vi "EOL All-Station AI Debug Buffer.vi"(5 "number of stations":i32=4, 7 "station idx":i32=4, 8 "Data to Write (Ch-Ro, Samp-Col)":sgl[][](array[numeric]) format="%.2f", 9 "Buffer Size (seconds/2500)":i32=5000, 11 "Mode":enum16{"Initialize", "Read", "Write"}(ring)=enum."Read") -> (2 "Data Read (Samp-Ro, Ch-Col)":sgl[][](array[numeric]) format="%.2f")   [LabVIEW 2018]
doc: "This VI is used in many locations throughout the program as a data buffer. It serves mainly two purposes. In alarms and logging, the DAQ data, whether scaled or voltage, is entered into the buffer. In other parts of the program, data is read from the buffer. Its length is based on the # of samples it was initialized to.\n\nA read will always return the latest data of the size requested."
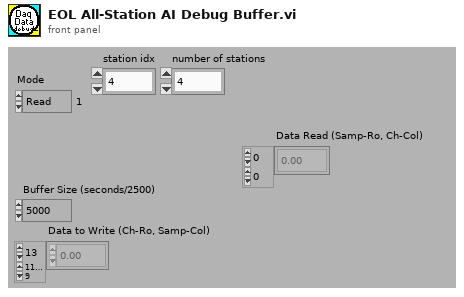
[diagram p1: front panel]
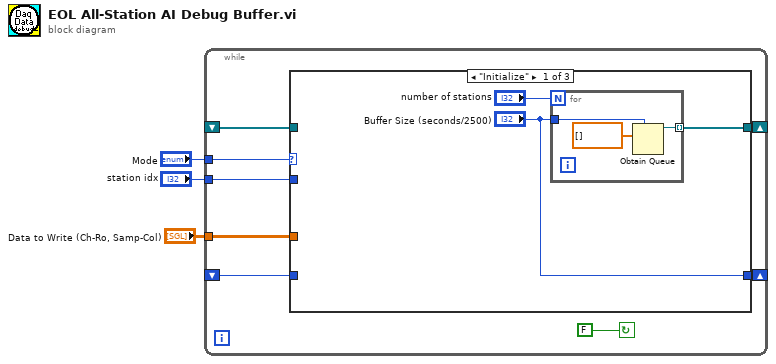
[diagram p0: block diagram]
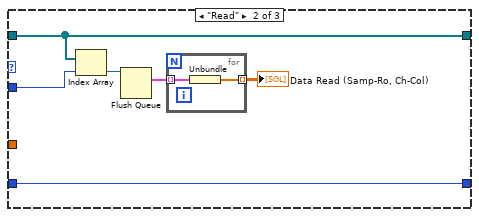
[diagram p2: hidden frame]
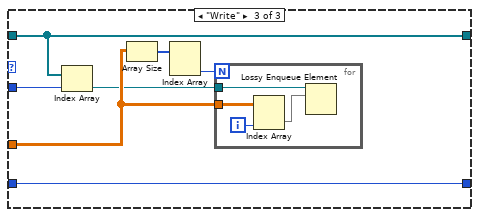
[diagram p3: hidden frame]
diagram:
  n1 = while {
    shift-left: _ -> [w11]
    shift-right: [w10] -> _
    tunnel: "Mode" -> [w8]
    tunnel: "station idx" -> [w7]
    tunnel: "Data to Write (Ch-Ro, Samp-Col)" -> [w6]
    shift-right: [w5] -> _
    shift-left: _ -> [w4]
    stop <- FALSE continue-if-true
    n2 = case shown="\"Initialize\"" w8 {
      tunnel: ["Buffer Size (seconds/2500)" w21 w32] -> w10
      tunnel: w11 -> [_ w21 w32]
      tunnel: w7 -> [_ w22 w31]
      tunnel: w6 -> [_ _ w30]
      tunnel: [w12 w20 w29] -> w5
      tunnel: w4 -> [_ w20 w29]
      frame "Initialize" {
        n3 = for {
          N: "number of stations" -> [_]
          tunnel: [w16] -> w12 mode=indexing
          tunnel: "Buffer Size (seconds/2500)" -> [w15]
          n4 = Obtain Queue(max queue size (-1, unlimited)=w15, element data type=sgl[] []) -> (queue out=w16:refnum<queue>)  [unwired: 3 in, 2 out]
        }
      }
      frame "Read" {
        n5 = Index Array(array=w20, index=w22) -> (element=w18:refnum<queue>)
        n6 = Flush Queue(queue=w18) -> (remaining elements=w19:cluster{sgl[]}[])  [unwired: 1 in, 2 out]
        n7 = for {
          tunnel: w19 -> [w25] mode=indexing
          tunnel: [w24] -> w23 mode=indexing
          n8 = Unbundle(w25) -> (w24:sgl[])
        }
        "Data Read (Samp-Ro, Ch-Col)" <- w23
      }
      frame "Write" {
        n9 = Index Array(array=w29, index=w31) -> (element=w26:refnum<queue>)
        n10 = Array Size(array=w30) -> (size(s)=w27:i32[])
        n11 = Index Array(array=w27) -> (element #2=w28:i32)  [unwired: 2 in, 1 out]
        n12 = for {
          N: w28 -> [_]
          tunnel: w26 -> [w36]
          tunnel: w30 -> [w35]
          i -> [w33]
          n13 = Index Array(array=w35, index (col)=w33) -> (element=w34:sgl[])  [unwired: 1 in]
          n14 = Lossy Enqueue Element(queue=w36, element=w34) -> ()  [unwired: 1 in, 4 out]
        }
      }
    }
  }
